vi "Get Proj Item Ref from Class Name.vi"(0 "ProjectI tem":refnum<vi>, 5 "Class Name":string, 11 "error in (no error)":errorcluster) -> (4 "Class Project Item Reference":refnum<vi>, 6 "Found":bool, 15 "error out":errorcluster)   [LabVIEW 2020, in "MVA Message Mapper.lvlib"]
uses:
  <vilib>/gpm_packages/@cs/Bus-message-mapper/Source/MVA Message Mapper.lvlib
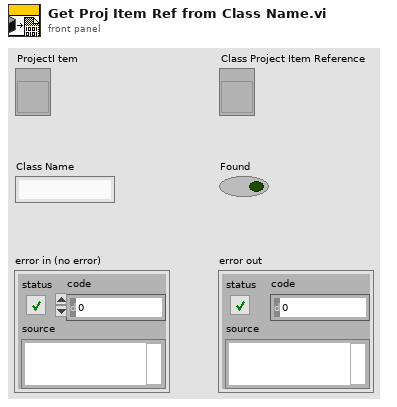
[diagram p1: front panel]
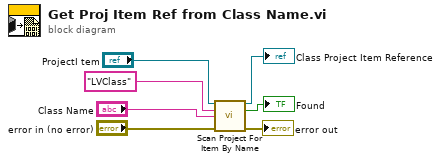
[diagram p0: block diagram]
diagram:
  n1 = call <vilib>:"Scan Project For Item By Name.vi"("ProjectItem in"="ProjectI tem", "Type"="LVClass", "Item Name"="Class Name", "error in (no error)"="error in (no error)") -> ("ProjectItem out"=→"Class Project Item Reference":refnum<vi>, "Found"=→"Found":bool, "error out"=→"error out":errorcluster)  [unwired: 9 in]
